vi "Items Double Click.vi"(4 "Row":i32, 6 "PlatMods":T1, 7 "Mods":cluster{"Double Click":bool, "Menu Key":bool}, 8 "error in (no error)":errorcluster, 9 "Button":u16, 10 "Coords":T2, 11 "Sequence Element in":refnum<class "Sequence Element.lvclass">) -> (0 "error out":errorcluster, 3 "Sequence Element out":refnum<class "Sequence Element.lvclass">)   [LabVIEW 2016, in "Sequence Element.lvclass"]
uses:
  Sequence Element.lvclass
  <vilib>/Utility/miscctls.llb/LVPoint32TypeDef.ctl
  Sequence Element.lvclass/Sequence Element.ctl
panel:
  out "Name":string
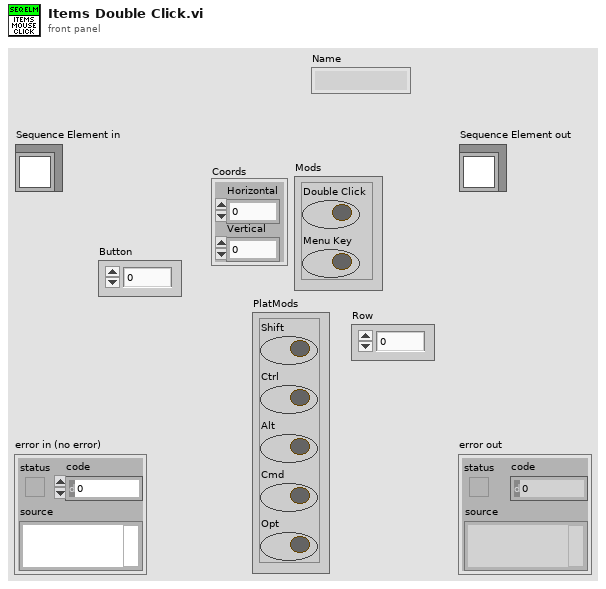
[diagram p1: front panel]
types:
  T1 = cluster{"Shift":bool, "Ctrl":bool, "Alt":bool, "Cmd":bool, "Opt":bool}
  T2 = typedef "LVPoint32TypeDef.ctl" = cluster{"Horizontal":i32, "Vertical":i32}
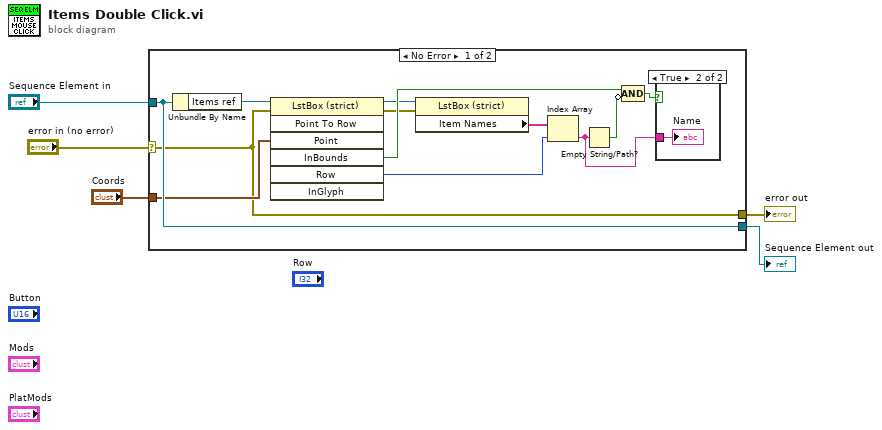
[diagram p0: block diagram]
diagram:
  n1 = case shown="No Error" "error in (no error)" {
    selector: "error in (no error)" -> [w14 w20]
    tunnel: [w14 w20] -> w4
    tunnel: [w17 w19] -> w2
    tunnel: "Sequence Element in" -> [w17 w19]
    tunnel: "Coords" -> [w15 _]
    frame No Error {
      n2 = Unbundle By Name(w17) -> ("Items ref"=w16:refnum<vi>)
      n3 = invoke class="LstBox (strict)" method="Point To Row"(reference=w16, error in=w14, "Point"=w15) -> (reference out=w11:refnum<vi>, error out=w10:errorcluster, "InBounds"=w13:bool, "Row"=w8:i32)  [unwired: 4 in, 3 out]
      n4 = property class="LstBox (strict)"(reference=w11, error in=w10) -> ("Item Names"=w9:string[])  [unwired: 2 out]
      n5 = Index Array(array=w9, index=w8) -> (element=w6:string)
      n6 = Empty String/Path?(string/path=w6) -> (empty?=w7:bool)
      n7 = Compound Arithmetic op=AND(w13, invert w7) -> (w12:bool)
      n8 = case shown="True" w12 {
        tunnel: w6 -> [_ w18]
        frame False {
        }
        frame True {
          "Name" <- w18
        }
      }
    }
    frame Error {
    }
  }
  "error out" <- w4
  "Sequence Element out" <- w2
